vi "Initialize Local Variable.vi"(8 "error in":errorcluster, 11 "Timed Node in":refnum<class "BLS Cycler Template.lvclass">) -> (0 "error out":errorcluster, 1 "Main to gRPC":T1, 2 "gRPC to Main":T2, 3 "Timed Node out":refnum<class "BLS Cycler Template.lvclass">)   [LabVIEW 2023, in "BLS Cycler Template.lvlib" / "BLS Cycler Template.lvclass"]
uses:
  BLS Cycler Template.lvclass
  Type Defs/gRPC to Main.ctl
  Type Defs/Main to gRPC.ctl
  BLS Cycler Template.lvclass/BLS Cycler Template.ctl
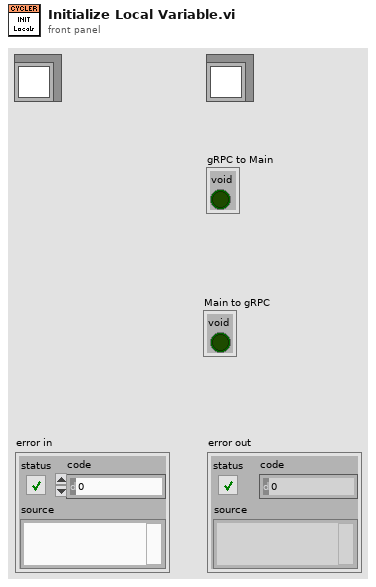
[diagram p1: front panel]
types:
  T1 = typedef "BLS Cycler Template.lvlib/BLS Cycler Template.lvclass/Main to gRPC.ctl" = cluster{"void":bool}
  T2 = typedef "BLS Cycler Template.lvlib/BLS Cycler Template.lvclass/gRPC to Main.ctl" = cluster{"void":bool}
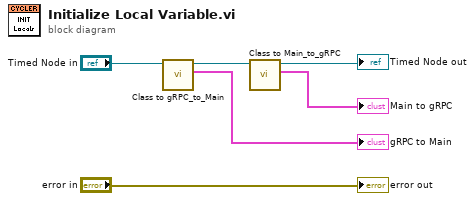
[diagram p0: block diagram]
diagram:
  n1 = call "Class to gRPC_to_Main.vi"("Timed Node in"="Timed Node in") -> ("gRPC to Main"=→"gRPC to Main":T2, "Timed Node out"=w5:refnum<class "BLS Cycler Template.lvclass">)  [unwired: 9 in]
  n2 = call "Class to Main_to_gRPC.vi"("Timed Node in"=w5) -> ("Main to gRPC"=→"Main to gRPC":T1, "Timed Node out"=→"Timed Node out":refnum<class "BLS Cycler Template.lvclass">)  [unwired: 9 in]
  "error out" <- "error in"
